vi "Ref saves data buffer.vi"(6 "Stop":bool, 7 "Initialise":bool, 11 "Array in":dbl[](array[numeric])) -> (1 "Save data":bool, 3 "Array out":dbl[][](array[numeric]))   [LabVIEW 2017]
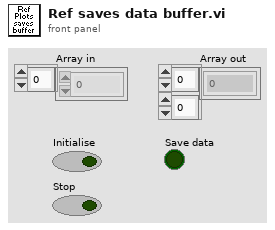
[diagram p1: front panel]
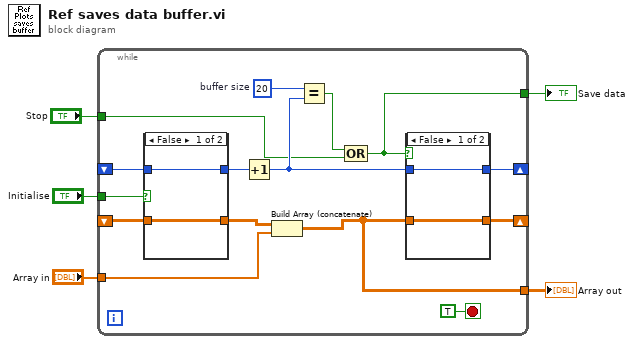
[diagram p0: block diagram]
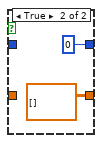
[diagram p2: hidden frame]
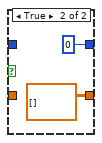
[diagram p3: hidden frame]
diagram:
  n1 = while {
    tunnel: "Array in" -> [w20]
    shift-right: [w11] -> _
    shift-left: _ -> [w17]
    shift-right: [w9] -> _
    shift-left: _ -> [w16]
    tunnel: [w10] -> w4
    tunnel: [w6] -> w3
    tunnel: "Initialise" -> [w13]
    tunnel: "Stop" -> [w7]
    stop <- TRUE stop-if-true
    w14 = 20  # buffer size
    n2 = case shown="False" w13 {
      tunnel: w17 -> [w26 _]
      tunnel: [w26 0] -> w18
      tunnel: w16 -> [w25 _]
      tunnel: [w25 dbl[][] []] -> w15
      frame False {
      }
      frame True {
      }
    }
    n3 = Increment(x=w18) -> (x+1=w12:i32)
    n4 = Build Array (concatenate)(w15, w20) -> (w10:dbl[][])
    n5 = Equal?(x=w14, y=w12) -> (x = y?=w8:bool)
    n6 = Compound Arithmetic op=OR(w8, w7) -> (w6:bool)
    n7 = case shown="False" w6 {
      tunnel: w12 -> [w22 _]
      tunnel: [w22 0] -> w11
      tunnel: w10 -> [w21 _]
      tunnel: [w21 dbl[][] []] -> w9
      frame False {
      }
      frame True {
      }
    }
  }
  "Array out" <- w4
  "Save data" <- w3
